vi "Control - Intake Air Desired MEP.vi"(0 "MEP Desired [bar]":sgl, 5 "Lambda Desired":sgl, 7 "AirMass Measured [mg/cyc] (optional)":sgl, 9 "Volumetric Efficiency [%]":sgl, 11 "Control Inputs":T1={"Engine Speed [RPM]"=0.0, "Engine Status"=enum."STALLED", "Load Control \nMode"=enum."High-Idle Governor", "dt(s)"=0.0, "Number of Cylinders"=0, "Engine Displacement [cc]"=0.0, "StoichAFR"=0.0, "Q.LHV Fuel [kJ/kg]"=0.0, "BattV PSU [V]"=0.0, "12V PSU [V]"=0.0, "5V PSU [V]"=0.0, "Pedal Position [%]"=0.0, "Oil Pressure [kPa]"=0.0, "Oil Temp [C]"=0.0, "Oil Level [%]"=0.0, "Engine Coolant Temp (ECT) [C]"=0.0, "Engine Coolant Pressure [kPa]"=0.0, "Rail Pressure [bar]"=0.0, "Fuel Pressure [kPa]"=0.0, "Fuel Temp [C]"=0.0, "Vacuum Pressure [kPa]"=0.0, "Throttle Position [%]"=0.0, "Cam1 Advance [CAD]"=0.0, "Cam2 Advance [CAD]"=0.0, "Cam3 Advance [CAD]"=0.0, "Cam4 Advance [CAD]"=0.0, "CA50 Control Output [CAD]"=[], "CA50 Control Output Valid"=[], "Intake Air Temp (IAT) [C]"=0.0, "Barometric Air Pressure [kPa]"=0.0, "Intake Air Rel. Humidity [%]"=0.0, "Mass Air Flow (MAF) [kg/hr]"=0.0, "Turbo Inlet Air Pressure [kPa]"=0.0, "Turbo Inlet Air Temp [C]"=0.0, "Turbo Outlet Air Pressure [kPa]"=0.0, "Turbo Outlet Air Temp [C]"=0.0, "CAC Outlet Pressure [kPa]"=0.0, "CAC Outlet Temp [C]"=0.0, "Intake Manifold Pressure (MAP) [kPa]"=0.0, "Intake Manifold Temp (MAT) [C]"=0.0, "Exhaust Manifold Pressure [kPa]"=0.0, "Exhaust Manifold Temp [C]"=0.0, "HighP EGR Cooler Outlet Pressure [kPa]"=0.0, "HighP EGR Cooler Outlet Temp [C]"=0.0, "HighP EGR Differential Pressure [kPa]"=0.0, "HighP EGR Valve Position [%]"=0.0, "Turbo Outlet Exhaust Pressure [kPa]"=0.0, "Turbo Outlet Exhaust Temp [C]"=0.0, "VGT Position 1 [%]"=0.0, "VGT Position 2 [%]"=0.0, "Turbo Speed 1 [RPM]"=0.0, "Turbo Speed 2 [RPM]"=0.0, "LowP EGR Differential Pressure [kPa]"=0.0, "LowP EGR Valve Position [%]"=0.0, "UEGO1Lambda"=0.0, "UEGO1_Hot"=FALSE, "UEGO2Lambda"=0.0, "UEGO2_Hot"=FALSE, "Knock Intensity"=[], "Knock"=[]} {"Knock Intensity" format="%.2f"; "CA50 Control Output [CAD]" format="%.2f"; "Exhaust Manifold Temp [C]" format="%#_6f"; "UEGO2Lambda" format="%.2f"; "Intake Manifold Temp (MAT) [C]" format="%#_6f"; "UEGO1Lambda" format="%.2f"}, 12 "MEP Measured [bar] (optional)":sgl) -> (10 "Air Mass Desired [mg/cyc]":sgl, 15 "Intake MAP Desired [kPa]":sgl)   [LabVIEW 2015, in "ECS-RT.lvlib"]
uses:
  ECS-RT.lvlib
  Typedefs/Control Inputs/Control Inputs.ctl
  Typedefs/EPT/Engine Status.ctl
  Typedefs/MISC/Load Control Mode.ctl
  ECS-Shared.lvlib
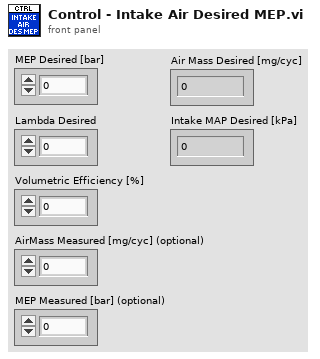
[diagram p1: front panel]
types:
  T1 = typedef "ECS-Shared.lvlib/Control Inputs.ctl" = cluster{"Engine Speed [RPM]":sgl, "Engine Status":T2, "Load Control \nMode":T3, "dt(s)":sgl, "Number of Cylinders":u8, "Engine Displacement [cc]":sgl, "StoichAFR":sgl, "Q.LHV Fuel [kJ/kg]":sgl, "BattV PSU [V]":sgl, "12V PSU [V]":sgl, "5V PSU [V]":sgl, "Pedal Position [%]":sgl, "Oil Pressure [kPa]":sgl, "Oil Temp [C]":sgl, "Oil Level [%]":sgl, "Engine Coolant Temp (ECT) [C]":sgl, "Engine Coolant Pressure [kPa]":sgl, "Rail Pressure [bar]":sgl, "Fuel Pressure [kPa]":sgl, "Fuel Temp [C]":sgl, "Vacuum Pressure [kPa]":sgl, "Throttle Position [%]":sgl, "Cam1 Advance [CAD]":sgl, "Cam2 Advance [CAD]":sgl, "Cam3 Advance [CAD]":sgl, "Cam4 Advance [CAD]":sgl, "CA50 Control Output [CAD]":sgl[], "CA50 Control Output Valid":bool[], "Intake Air Temp (IAT) [C]":sgl, "Barometric Air Pressure [kPa]":sgl, "Intake Air Rel. Humidity [%]":sgl, "Mass Air Flow (MAF) [kg/hr]":sgl, "Turbo Inlet Air Pressure [kPa]":sgl, "Turbo Inlet Air Temp [C]":sgl, "Turbo Outlet Air Pressure [kPa]":sgl, "Turbo Outlet Air Temp [C]":sgl, "CAC Outlet Pressure [kPa]":sgl, "CAC Outlet Temp [C]":sgl, "Intake Manifold Pressure (MAP) [kPa]":sgl, "Intake Manifold Temp (MAT) [C]":sgl, "Exhaust Manifold Pressure [kPa]":sgl, "Exhaust Manifold Temp [C]":sgl, "HighP EGR Cooler Outlet Pressure [kPa]":sgl, "HighP EGR Cooler Outlet Temp [C]":sgl, "HighP EGR Differential Pressure [kPa]":sgl, "HighP EGR Valve Position [%]":sgl, "Turbo Outlet Exhaust Pressure [kPa]":sgl, "Turbo Outlet Exhaust Temp [C]":sgl, "VGT Position 1 [%]":sgl, "VGT Position 2 [%]":sgl, "Turbo Speed 1 [RPM]":sgl, "Turbo Speed 2 [RPM]":sgl, "LowP EGR Differential Pressure [kPa]":sgl, "LowP EGR Valve Position [%]":sgl, "UEGO1Lambda":sgl, "UEGO1_Hot":bool, "UEGO2Lambda":sgl, "UEGO2_Hot":bool, "Knock Intensity":sgl[], "Knock":bool[]}
  T2 = typedef "ECS-Shared.lvlib/Engine Status.ctl" = enum16{"OFF", "STALLED", "CRANKING", "RUNNING", "ACCEL", "DECEL", "SAFE"}
  T3 = typedef "ECS-Shared.lvlib/Load Control Mode.ctl" = enum16{"No Governor", "Low-Idle Governor", "High-Idle Governor"}
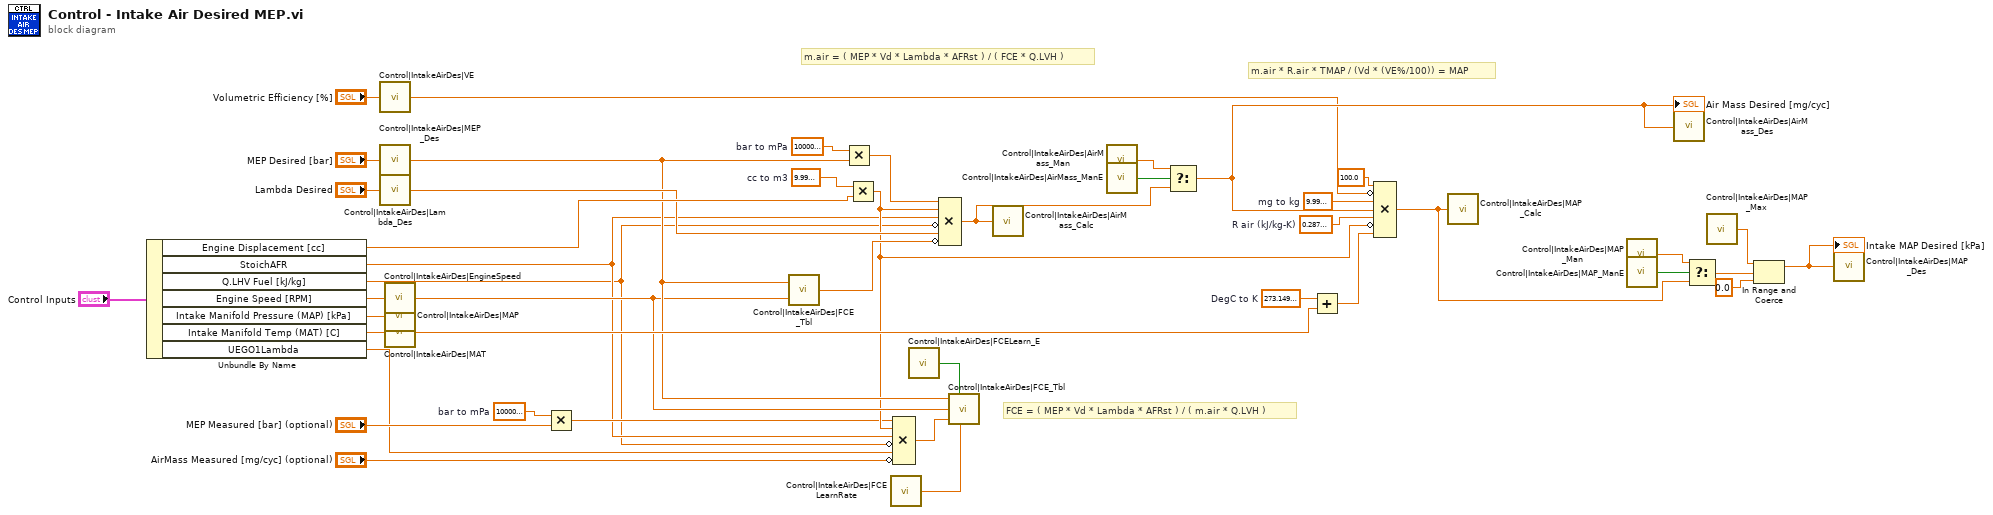
[diagram p0: block diagram]
diagram:
  w7 = sgl 100000000.0  # bar to mPa
  w24 = sgl 1e-06  # mg to kg
  w21 = sgl 273.15  # DegC to K
  w22 = sgl 0.287  # R air (kJ/kg-K)
  w16 = sgl 100000000.0  # bar to mPa
  w15 = sgl 1e-06  # cc to m3
  # "FCE = ( MEP * Vd * Lambda * AFRst ) / ( m.air * Q.LVH )"
  # "m.air * R.air * TMAP / (Vd * (VE%/100)) = MAP"
  # "m.air = ( MEP * Vd * Lambda * AFRst ) / ( FCE * Q.LVH )"
  n1 = Unbundle By Name("Control Inputs") -> ("Engine Displacement [cc]"=w28:sgl, "StoichAFR"=w4:sgl, "Q.LHV Fuel [kJ/kg]"=w3:sgl, "Engine Speed [RPM]"=w12:sgl, "Intake Manifold Pressure (MAP) [kPa]"=w31:sgl, "Intake Manifold Temp (MAT) [C]"=w29:sgl, "UEGO1Lambda"=w1:sgl)
  n2 = call "Control|IntakeAirDes|VE"("Value"="Volumetric Efficiency [%]") -> ()
  n3 = call "Control|IntakeAirDes|MEP_Des"("Value"="MEP Desired [bar]") -> ()
  n4 = call "Control|IntakeAirDes|Lambda_Des"("Value"="Lambda Desired") -> ()
  n5 = call "Control|IntakeAirDes|EngineSpeed"("Value"=w12) -> ()
  n6 = call "Control|IntakeAirDes|MAP"("Value"=w31) -> ()
  n7 = call "Control|IntakeAirDes|MAT"("Value"=w29) -> ()
  n8 = Multiply(x=w7, y="MEP Measured [bar] (optional)") -> (x*y=w5:sgl)
  n9 = call "Control|IntakeAirDes|FCE_Tbl"("Y Index"=w12, "X Index"="MEP Desired [bar]") -> ("Z"=w17:sgl)
  n10 = Multiply(x=w16, y="MEP Desired [bar]") -> (x*y=w25:sgl)
  n11 = Multiply(x=w15, y=w28) -> (x*y=w8:sgl)
  n12 = call "Control|IntakeAirDes|FCELearnRate"() -> ("Value"=w9:sgl)
  n13 = Compound Arithmetic op=MULTIPLY(w5, w8, w4, invert w3, w1, invert "AirMass Measured [mg/cyc] (optional)") -> (w10:sgl)
  n14 = call "Control|IntakeAirDes|FCELearn_E"() -> ("Value"=w11:bool)
  n15 = Compound Arithmetic op=MULTIPLY(w25, w8, w4, invert w3, "Lambda Desired", invert w17) -> (w20:sgl)
  n16 = call "Control|IntakeAirDes|FCE_Tbl"("X"="MEP Desired [bar]", "Adapt"=w11, "Y"=w12, "Z"=w10, "%/100"=w9) -> ()  [unwired: 1 in]
  n17 = call "Control|IntakeAirDes|AirMass_Calc"("Value"=w20) -> ()
  n18 = call "Control|IntakeAirDes|AirMass_Man"() -> ("Value"=w18:sgl)
  n19 = call "Control|IntakeAirDes|AirMass_ManE"() -> ("Value"=w19:bool)
  n20 = Select(t=w18, s=w19, f=w20) -> (s? t:f=w33:sgl)
  "Air Mass Desired [mg/cyc]" <- w33
  n21 = Add(x=w21, y=w29) -> (x+y=w23:sgl)
  n22 = Compound Arithmetic op=MULTIPLY(sgl 100.0 ("value"), invert "Volumetric Efficiency [%]", w24, w33, w22, invert w8, w23) -> (w32:sgl)
  n23 = call "Control|IntakeAirDes|MAP_Calc"("Value"=w32) -> ()
  n24 = call "Control|IntakeAirDes|MAP_Man"() -> ("Value"=w35:sgl)
  n25 = call "Control|IntakeAirDes|MAP_ManE"() -> ("Value"=w36:bool)
  n26 = call "Control|IntakeAirDes|AirMass_Des"("Value"=w33) -> ()
  n27 = Select(t=w35, s=w36, f=w32) -> (s? t:f=w34:sgl)
  n28 = call "Control|IntakeAirDes|MAP_Max"() -> ("Value"=w38:sgl)
  n29 = In Range and Coerce(upper limit=w38, x=w34, lower limit=sgl 0.0) -> (coerced(x)=w37:sgl)  [unwired: 1 out]
  "Intake MAP Desired [kPa]" <- w37
  n30 = call "Control|IntakeAirDes|MAP_Des"("Value"=w37) -> ()
